vi "Read.vi"(8 "error in (no error)":errorcluster, 9 "Timeout ms (1000)":i32=1000, 11 "WebSocket Client in":refnum<class "WebSocket Client.lvclass">) -> (0 "error out":errorcluster, 1 "Format":T1, 2 "Payload":string, 3 "WebSocket Client out":refnum<class "WebSocket Client.lvclass">)   [LabVIEW 2020, in "HTTP Server.lvlib" / "WebSocket Client.lvclass"]
uses:
  WebSocket Client.lvclass
  WebSocket Format.ctl
  Lock Type.ctl
  WebSocket Client.lvclass/WebSocket Client.ctl
  HTTP Server.lvlib
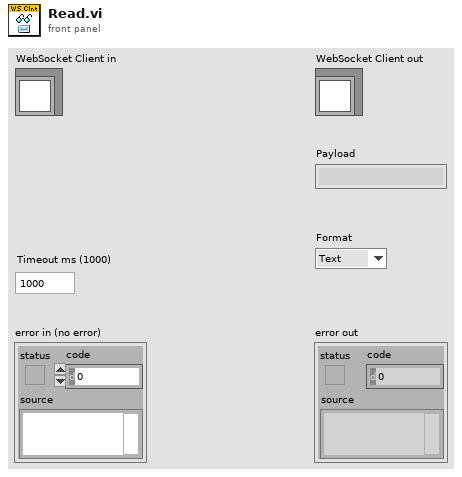
[diagram p1: front panel]
types:
  T1 = typedef "HTTP Server.lvlib/WebSocket Format.ctl" = enum16{"Text", "Binary"}
  T2 = typedef "HTTP Server.lvlib/WebSocket Client.lvclass/Lock Type.ctl" = enum16{"Read", "Write"}
  T3 = typedef "HTTP Server.lvlib/WebSocket Client.lvclass/Message Frame.ctl" = cluster{"FIN":bool, "RSV1":bool, "RSV2":bool, "RSV3":bool, "MASK":bool, "OpCode":T4, "Length":u64, "MaskingKey":u8[], "Payload":string}
  T4 = typedef "HTTP Server.lvlib/WebSocket Client.lvclass/OpCode.ctl" = enum8{"Continuation", "Text", "Binary", "Reserved3", "Reserved4", "Reserved5", "Reserved6", "Reserved7", "Close", "Ping", "Pong", "ReservedB", "ReservedC", "ReservedD", "ReservedE", "ReservedF"}
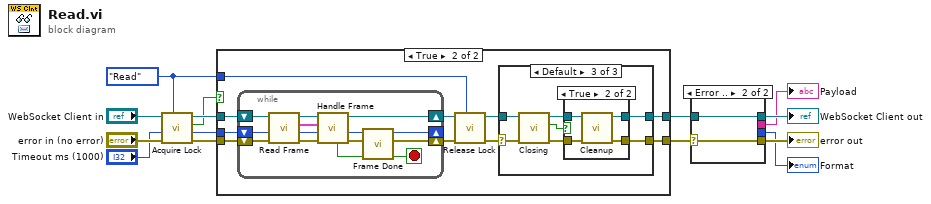
[diagram p0: block diagram]
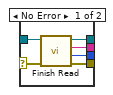
[diagram p2: hidden frame]
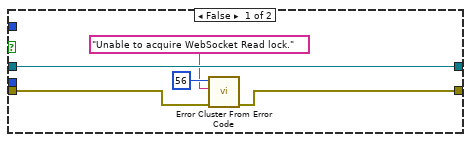
[diagram p3: hidden frame]
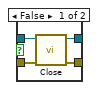
[diagram p6: hidden frame]
diagram:
  w8 = Lock_Type."Read" ("Lock Type")
  n1 = call "Acquire Lock.vi"("Lock Type"=w8, "error in (no error)"="error in (no error)", "Timeout ms"="Timeout ms (1000)", "WebSocket Client in"="WebSocket Client in") -> ("error out"=w13:errorcluster, "Remaining  Timeout"=w9:i32, "Acquired"=w1:bool, "WebSocket Client out"=w10:refnum<class "WebSocket Client.lvclass">)  [unwired: 4 in]
  n2 = case shown="True" w1 {
    tunnel: w10 -> [w19 w28]
    tunnel: w9 -> [_ w27]
    tunnel: w8 -> [_ w24]
    tunnel: [w17 w21] -> w7
    tunnel: [w19 w20] -> w5
    tunnel: w13 -> [w18 w29]
    frame False {
      n3 = call <vilib>:"Error Cluster From Error Code.vi"("error in (no error)"=w18, "error message (\"\")"="Unable to acquire WebSocket Read lock.", "error code (0)"=56) -> ("error out"=w17:errorcluster)  [unwired: 6 in]
    }
    frame True {
      n4 = while {
        shift-right: [w52] -> w26
        shift-left: w29 -> [w62]
        shift-right: [w57] -> w25
        shift-left: w28 -> [w60]
        shift-right: [w49] -> _
        shift-left: w27 -> [w59]
        stop <- w50 stop-if-true
        n5 = call "Read Frame.vi"("error in (no error)"=w62, "Timeout ms"=w59, "WebSocket Client in"=w60) -> ("error out"=w61:errorcluster, "Remaining  Timeout"=w55:i32, "Message Frame"=w56:T3, "WebSocket Client out"=w58:refnum<class "WebSocket Client.lvclass">)  [unwired: 5 in]
        n6 = call "Handle Frame.vi"("error in (no error)"=w61, "Timeout ms"=w55, "Message Frame"=w56, "WebSocket Client in"=w58) -> ("error out"=w54:errorcluster, "Remaining  Timeout"=w53:i32, "WebSocket Client out"=w57:refnum<class "WebSocket Client.lvclass">, "Complete"=w51:bool)  [unwired: 4 in]
        n7 = call "Frame Done.vi"("Payload Complete"=w51, "error in (no error)"=w54, "Timeout ms"=w53) -> ("Done"=w50:bool, "error out"=w52:errorcluster, "Remaining  Timeout"=w49:i32)  [unwired: 6 in]
      }
      n8 = call "Release Lock.vi"("Lock Type"=w24, "error in (no error)"=w26, "WebSocket Client in"=w25) -> ("error out"=w23:errorcluster, "WebSocket Client out"=w22:refnum<class "WebSocket Client.lvclass">)  [unwired: 7 in]
      n9 = case shown="Default" w23 {
        selector: w23 -> [w30 w33 w39]
        tunnel: w22 -> [w31 w32 w40]
        tunnel: [w30 w33 w34] -> w21
        tunnel: [w31 w32 w35] -> w20
        frame No Error {
        }
        frame Error {
        }
        frame Default {
          n10 = call "Closing.vi"("error in (no error)"=w39, "WebSocket Client in"=w40) -> ("error out"=w38:errorcluster, "Closing"=w37:bool, "WebSocket Client out"=w36:refnum<class "WebSocket Client.lvclass">)  [unwired: 7 in]
          n11 = case shown="True" w37 {
            tunnel: w38 -> [w44 w47]
            tunnel: w36 -> [w43 w48]
            tunnel: [w42 w45] -> w35
            tunnel: [w41 w46] -> w34
            frame False {
              n12 = call "Close.vi"("error in (no error)"=w44, "WebSocket Client in"=w43) -> ("error out"=w41:errorcluster, "WebSocket Client out"=w42:refnum<class "WebSocket Client.lvclass">)  [unwired: 8 in]
            }
            frame True {
              n13 = call "Cleanup.vi"("error in (no error)"=w47, "WebSocket Client in"=w48) -> ("error out"=w46:errorcluster, "WebSocket Client out"=w45:refnum<class "WebSocket Client.lvclass">)  [unwired: 8 in]
            }
          }
        }
      }
    }
  }
  n14 = case shown="Error .." w7 {
    selector: w7 -> [w68 w69]
    tunnel: [w67 w69] -> w6
    tunnel: w5 -> [w66 w70]
    tunnel: [w65 w70] -> w4
    tunnel: [w64 _] -> w3
    tunnel: [w63 _] -> w2
    frame No Error {
      n15 = call "Finish Read.vi"("error in (no error)"=w68, "WebSocket Client in"=w66) -> ("error out"=w67:errorcluster, "Format"=w63:T1, "Payload"=w64:string, "WebSocket Client out"=w65:refnum<class "WebSocket Client.lvclass">)  [unwired: 6 in]
    }
    frame Error {
    }
  }
  "error out" <- w6
  "WebSocket Client out" <- w4
  "Payload" <- w3
  "Format" <- w2
